vi "Tank_oneC.vi"   [LabVIEW 2012, in "Serenity_mk2.lvrbt"]
uses:
  Serenity_mk2.lvrbt
  <vilib>/NXT/Hardware/Plugins/Tetrix 180 deg Servo/Tetrix180ServoAddress.ctl
  <vilib>/NXT/Hardware/Plugins/Tetrix DC Motor/TetrixDCMotorAddress.ctl
  <vilib>/NXT/NXTIO Xnodes/NXTIONodeSubVIs/TETRIX IO Move Servos.vi
  <vilib>/FTC/FTC Calculate Drive Power - Tank.vi
  <vilib>/NXT/NXTIO Xnodes/NXTIONodeSubVIs/TETRIX IO Move DC Motors.vi
  <vilib>/NXT/NXTIO Xnodes/NXTIONodeSubVIs/TETRIX IO Check Battery.vi
  <vilib>/NXT/NXTIO Xnodes/NXTIONodeSubVIs/TETRIX IO Stop DC Motors.vi
  <vilib>/NXT/NXTIO Xnodes/AddressXNode/NXTIOAddress.xnode
  <vilib>/NXT/Subs/LVHSConnector.ctl
  <vilib>/NXT/NXTIO Xnodes/NXTIOXNode/NXTIO.xnode
  MecanumDrive/Mecanum Drive.lvrbt
  <vilib>/NXT/LegoClasses/BrickReference/BrickReference.lvclass
panel:
  # "This VI was generated based on your configuration in the Remote Control Editor. You may modify the code as needed for your robot. To test this program for an FTC match, return to the Remote Control Editor, select the \"Run Program\" tab, and choose \"Teleop\"."
types:
  T1 = typedef "Tetrix180ServoAddress.ctl" = i32
  T2 = typedef "LVHSConnector.ctl" = refnum<class "BrickReference.lvclass">
  T3 = typedef "TetrixDCMotorAddress.ctl" = i32
  T4 = cluster{"TetrixDCMotor":T3, "TetrixDCMotor 2":T3}
  T5 = typedef "FTC ControllerState.ctl" = cluster{"Left X":i8, "Left Y":i8, "Right X":i8, "Right Y":i8, "Button Encoding 9-12":u8, "Button Encoding 1-8":u8, "POV":T6}
  T6 = typedef "FTC POVState.ctl" = i8
  T7 = typedef "FTC ButtonEventType.ctl" = enum16{"Pressed", "Released"}
  T8 = cluster{"Button ID":enum16{"None", "Button 1", "Button 2", "Button 3", "Button 4", "Button 5", "Button 6", "Button 7", "Button 8", "Button 9", "Button 10", "Button 11", "Button 12", "POV Up", "POV Up Right", "POV Right", "POV Down Right", "POV Down", "POV Down Left", "POV Left", "POV Up Left"}, "Event Type":T7}[]
  T9 = typedef "FTC ButtonState.ctl" = cluster{"Button 1":bool, "Button 2":bool, "Button 3":bool, "Button 4":bool, "Button 5":bool, "Button 6":bool, "Button 7":bool, "Button 8":bool, "Button 9":bool, "Button 10":bool, "Button 11":bool, "Button 12":bool, "POV":T6}
  T10 = enum16{"None", "Button 1", "Button 2", "Button 3", "Button 4", "Button 5", "Button 6", "Button 7", "Button 8", "Button 9", "Button 10", "Button 11", "Button 12", "POV Up", "POV Up Right", "POV Right", "POV Down Right", "POV Down", "POV Down Left", "POV Left", "POV Up Left"}
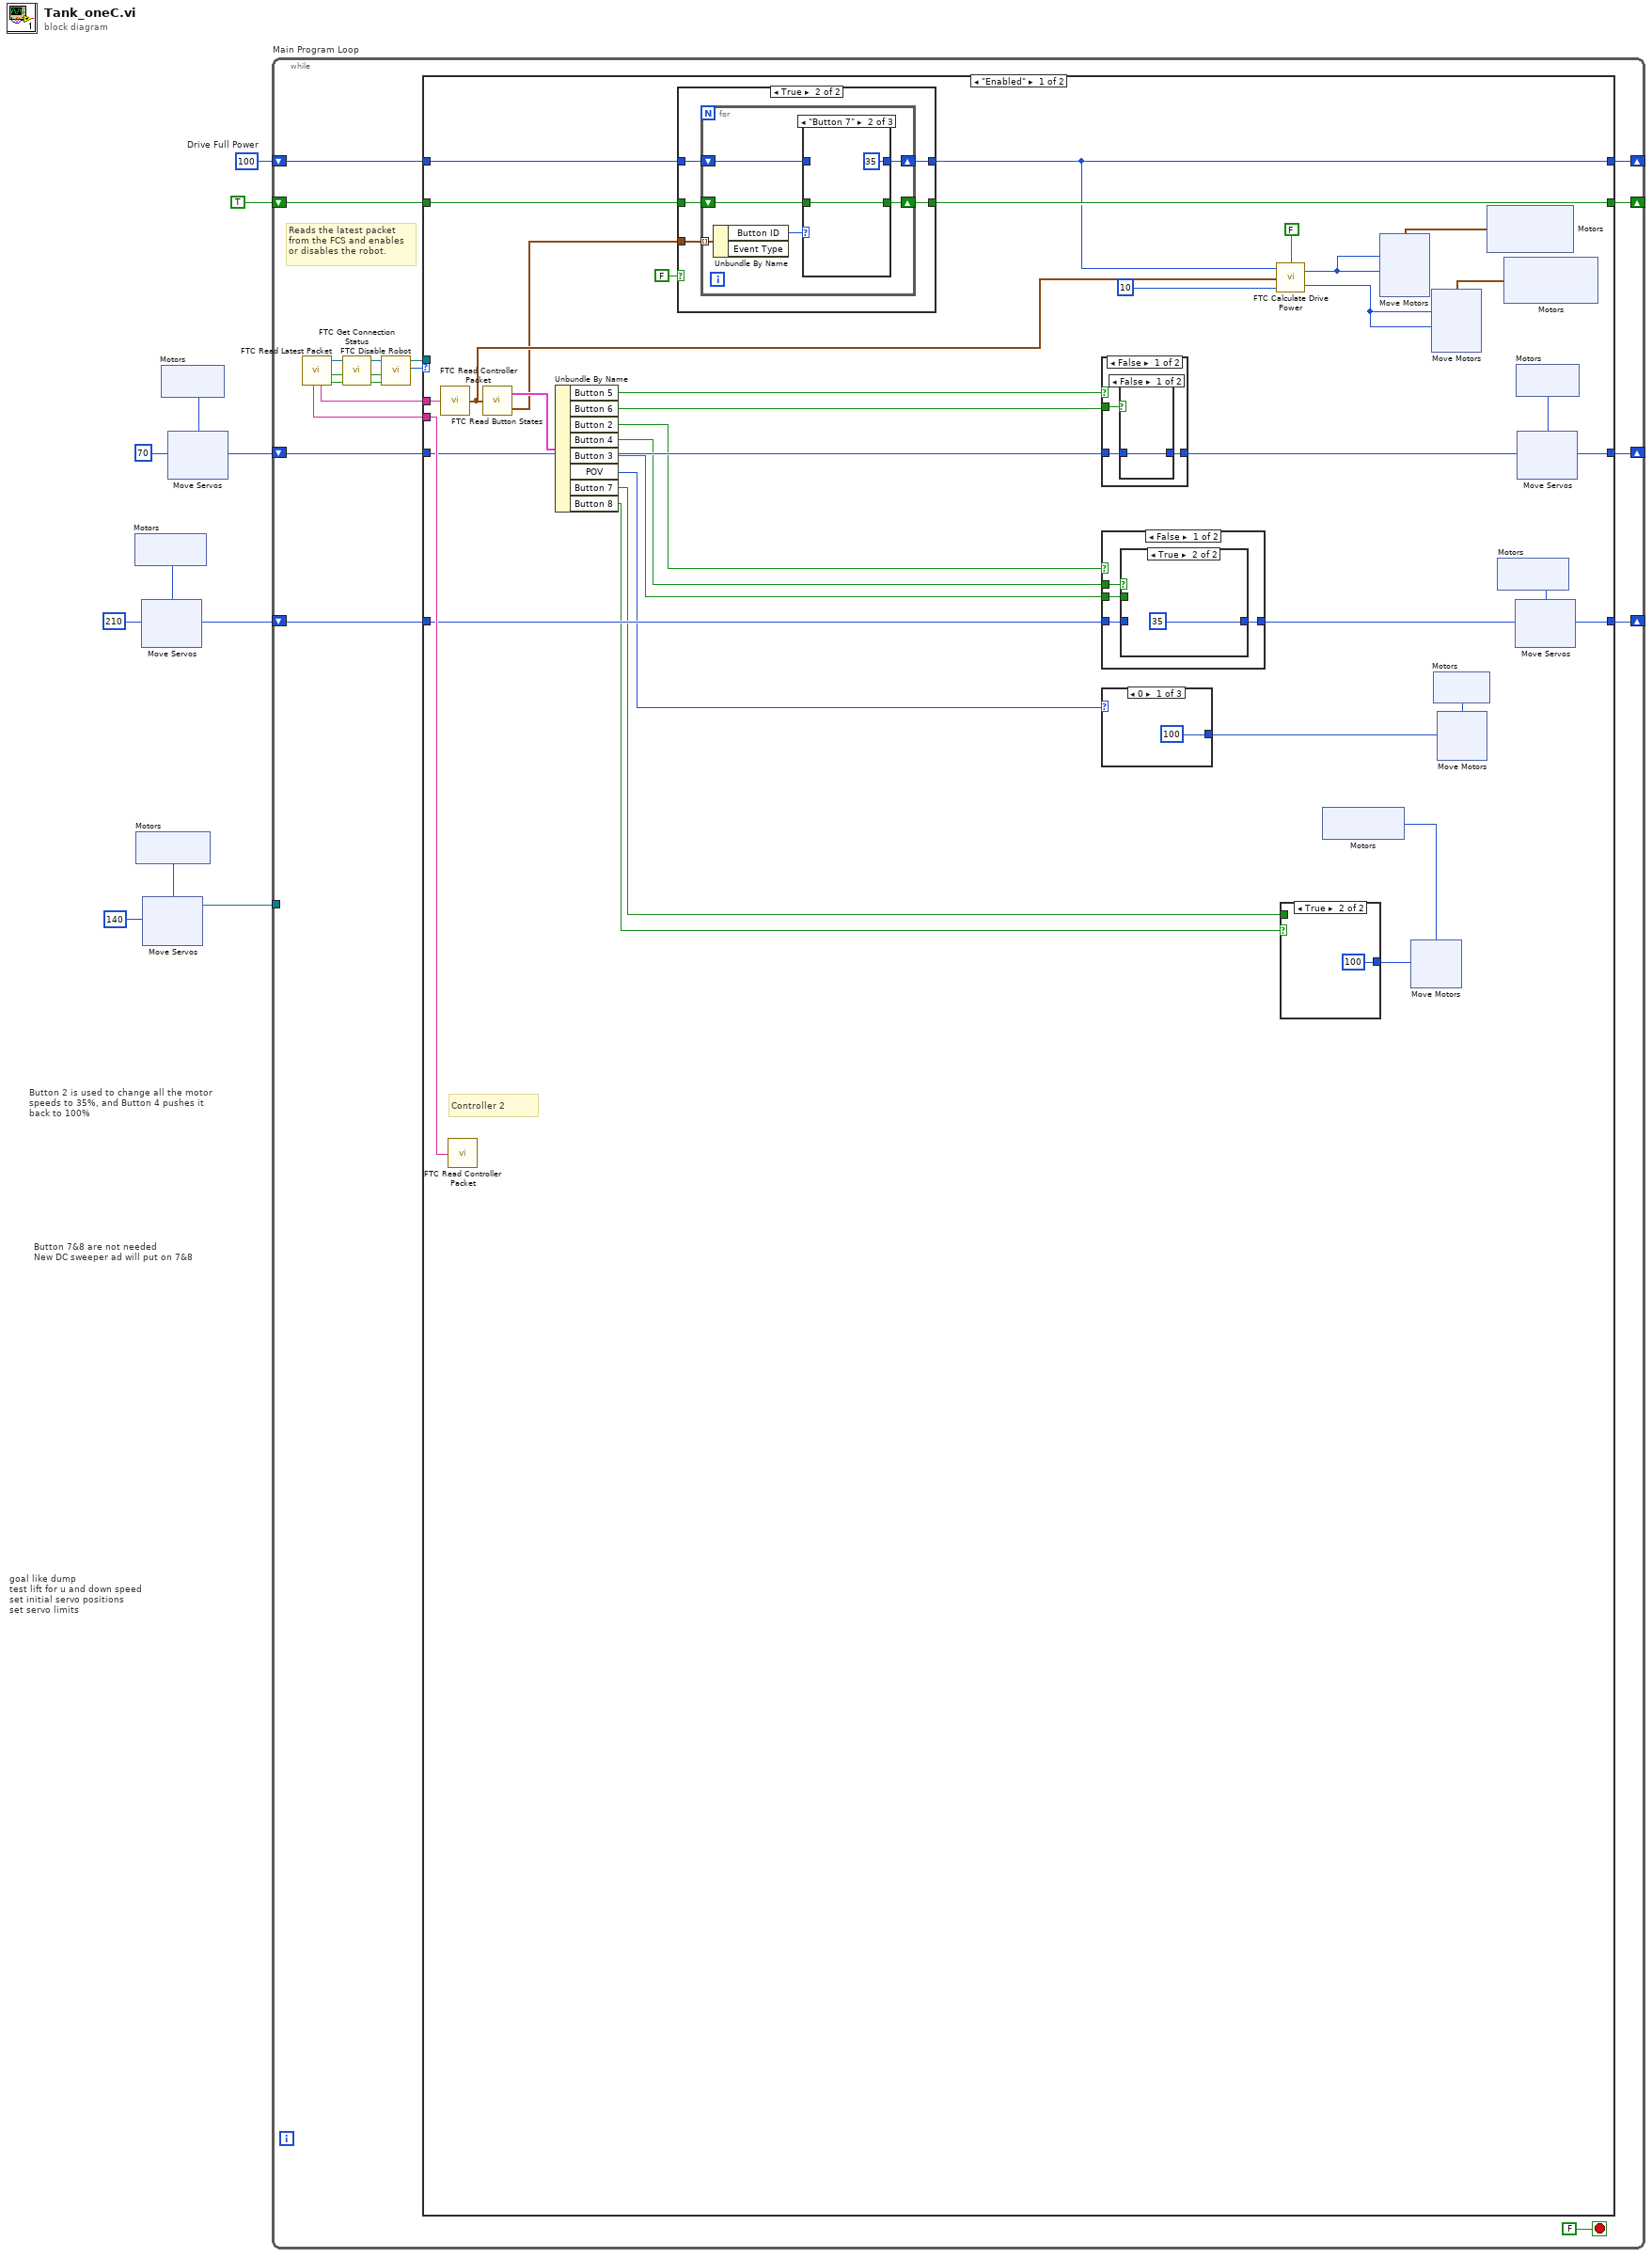
[diagram p0: block diagram]
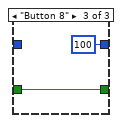
[diagram p4: hidden frame]
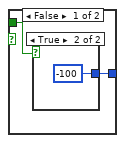
[diagram p5: hidden frame]
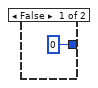
[diagram p6: hidden frame]
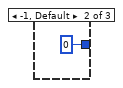
[diagram p7: hidden frame]
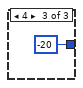
[diagram p8: hidden frame]
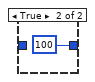
[diagram p9: hidden frame]
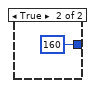
[diagram p10: hidden frame]
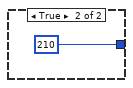
[diagram p12: hidden frame]
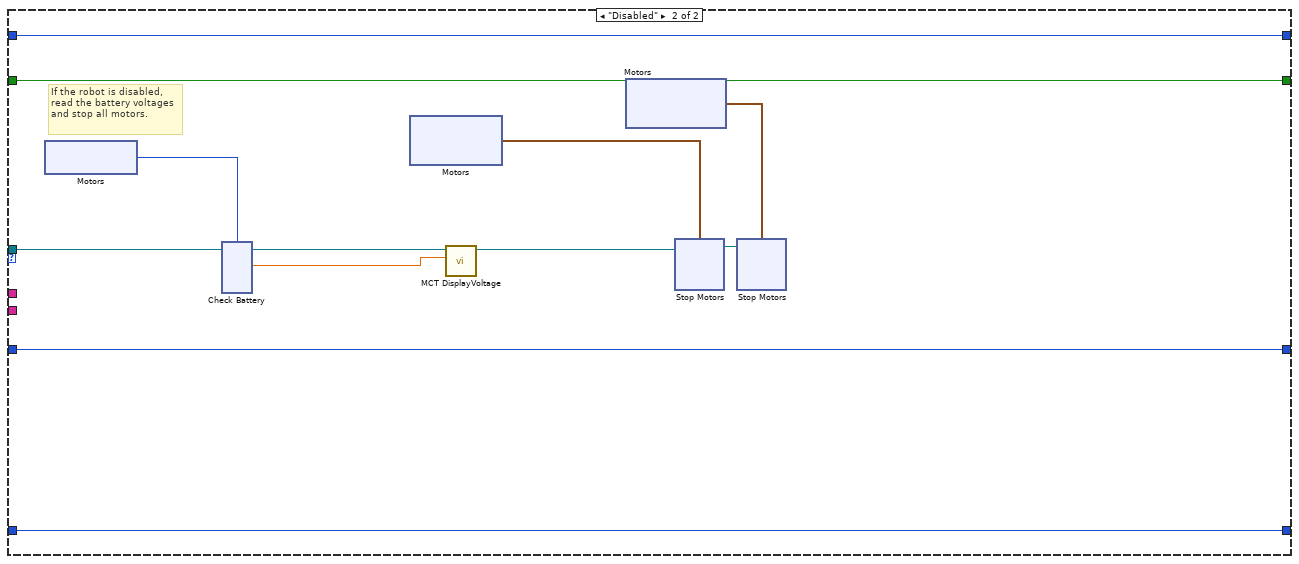
[diagram p13: hidden frame]
diagram:
  w4 = u8 210 ("Position 1")
  w6 = u8 70 ("Position 1")
  w9 = i8 100  # Drive Full Power
  # "Button 2 is used to change all the motor \nspeeds to 35%, and Button 4 pushes it \nback to 100%"
  # "goal like dump\ntest lift for u and down speed\nset initial servo positions\nset servo limits"
  # "Button 7&8 are not needed\nNew DC sweeper ad will put on 7&8"
  n1 = xnode "Motors"() -> ("Motor"=w5:T1)
  n2 = xnode "Motors"() -> ("Motor"=w3:T1)
  n3 = xnode "Move Servos"("Position 1"=w4, "Motors"=w5) -> ()  [unwired: 1 in, 1 out]
  n4 = xnode "Move Servos"("Position 1"=u8 140, "Motors"=w3) -> ("NXT/EV3"=w1:T2)  [unwired: 1 in]
  n5 = xnode "Motors"() -> ("Motor"=w7:T1)
  n6 = xnode "Move Servos"("Position 1"=w6, "Motors"=w7) -> ()  [unwired: 1 in, 1 out]
  n7 = while "Main Program Loop" {
    shift-right: [w16] -> _
    shift-left: w9 -> [w17]
    shift-right: [w14] -> _
    shift-left: TRUE -> [w15]
    shift-right: [w13] -> _
    shift-left: w6 -> [w12]
    shift-right: [w11] -> _
    shift-left: w4 -> [w10]
    tunnel: w1 -> [_]
    stop <- FALSE stop-if-true
    # "Reads the latest packet\nfrom the FCS and enables\nor disables the robot."
    n8 = call <vilib>:"FTC Read Latest Packet.vi"() -> ("Packet Received?"=w25:bool, "Stopped?"=w22:bool, "NXT"=w24:T2, "Controller 1"=w27:string, "Controller 2"=w26:string)  [unwired: 6 in, 1 out]
    n9 = call <vilib>:"FTC Get Connection Status.vi"("Packet Received?"=w25, "Stopped?"=w22, "NXT"=w24) -> ("Online?"=w19:bool, "Stopped?"=w20:bool, "NXT"=w21:T2)  [unwired: 5 in]
    n10 = call <vilib>:"FTC Disable Robot.vi"("Online?"=w19, "Stopped?"=w20, "NXT"=w21) -> ("Enabled?"=w23:enum16{"Disabled", "Enabled"}, "NXT"=w18:T2)  [unwired: 3 in]
    n11 = case "disableCase" shown="\"Enabled\"" w23 {
      tunnel: w27 -> [w62 _]
      tunnel: w26 -> [w61 _]
      tunnel: w18 -> [_ w164]
      tunnel: w17 -> [w60 w156]
      tunnel: [w50 w156] -> w16
      tunnel: w15 -> [w59 w155]
      tunnel: [w58 w155] -> w14
      tunnel: [w41 w154] -> w13
      tunnel: w12 -> [w42 w154]
      tunnel: [w46 w153] -> w11
      tunnel: w10 -> [w45 w153]
      frame "Enabled" {
        # "Controller 2"
        n12 = call <vilib>:"FTC Read Controller Packet.vi"("Packet"=w62) -> ("Controller State"=w48:T5)  [unwired: 4 in]
        n13 = call <vilib>:"FTC Read Controller Packet.vi"("Packet"=w61) -> ()  [unwired: 4 in, 1 out]
        n14 = call <vilib>:"FTC Read Button States.vi"("Controller State"=w48) -> ("Button Events"=w30:T8, "Button States"=w56:T9)  [unwired: 2 in]
        n15 = Unbundle By Name(w56) -> ("Button 5"=w44:bool, "Button 6"=w43:bool, "Button 2"=w37:bool, "Button 4"=w38:bool, "Button 3"=w39:bool, "POV"=w40:T6, "Button 7"=w32:bool, "Button 8"=w31:bool)
        n16 = case shown="True" FALSE {
          tunnel: w60 -> [w64 w69]
          tunnel: w59 -> [w63 w68]
          tunnel: [w63 w67] -> w58
          tunnel: [w64 w66] -> w50
          tunnel: w30 -> [_ w65]
          frame False {
          }
          frame True {
            n17 = for {
              tunnel: w65 -> [w75] mode=indexing
              shift-right: [w70] -> w66
              shift-left: w69 -> [w73]
              shift-right: [w71] -> w67
              shift-left: w68 -> [w72]
              n18 = Unbundle By Name(w75) -> ("Button ID"=w74:T10)  [unwired: 1 out]
              n19 = case shown="\"Button 7\"" w74 {
                tunnel: w73 -> [w76 _ _]
                tunnel: w72 -> [w77 w78 w80]
                tunnel: [w77 w78 w80] -> w71
                tunnel: [w76 i8 35 i8 100] -> w70
                frame "None", Default {
                }
                frame "Button 7" {
                }
                frame "Button 8" {
                }
              }
            }
          }
        }
        n20 = case shown="False" w44 {
          tunnel: w43 -> [w106 _]
          tunnel: w42 -> [w107 _]
          tunnel: [w108 u8 160 ("Position 1")] -> w41
          frame False {
            n21 = case shown="False" w106 {
              tunnel: [w109 u8 100 ("lower limit")] -> w108
              tunnel: w107 -> [w109 _]
              frame False {
              }
              frame True {
              }
            }
          }
          frame True {
          }
        }
        n22 = case shown="False" w37 {
          tunnel: w38 -> [w115 _]
          tunnel: [w114 u8 210] -> w46
          tunnel: w45 -> [w113 _]
          tunnel: w39 -> [w112 _]
          frame False {
            n23 = case shown="True" w115 {
              tunnel: [w116 u8 35] -> w114
              tunnel: w113 -> [w116 _]
              tunnel: w112 -> [_ _]
              frame False {
              }
              frame True {
              }
            }
          }
          frame True {
          }
        }
        n24 = case shown="0" w40 {
          tunnel: [i8 100 ("Power/Speed 1") i8 0 ("Power/Speed 1") i8 -20 ("Power/Speed 1")] -> w35
          frame 0 {
          }
          frame -1, Default {
          }
          frame 4 {
          }
        }
        n25 = call-poly <vilib>:"FTC Calculate Drive Power.vi"("Reverse"=FALSE, "Deadband (10)"=i8 10, "Controller State"=w48, "Power Level (50)"=w50) -> ("Right Motor Power"=w49:i8, "Left Motor Power"=w51:i8)
        n26 = case shown="True" w31 {
          tunnel: w32 -> [w91 _]
          tunnel: [w90 i8 100] -> w34
          frame False {
            n27 = case shown="True" w91 {
              tunnel: [i8 0 i8 -100] -> w90
              frame False {
              }
              frame True {
              }
            }
          }
          frame True {
          }
        }
        n28 = xnode "Motors"() -> ("Motor"=w33:T3)
        n29 = xnode "Move Motors"("Power/Speed 1"=w34, "Motors"=w33) -> ()  [unwired: 1 in, 1 out]
        n30 = xnode "Motors"() -> ("Motor"=w36:T3)
        n31 = xnode "Move Motors"("Power/Speed 1"=w35, "Motors"=w36) -> ()  [unwired: 1 in, 1 out]
        n32 = xnode ("Motors")() -> ("Motor"=w52:cluster{"TetrixDCMotor":T3, "TetrixDCMotor":T3})
        n33 = xnode ("Move Motors")("Power/Speed 2"=w51, "Power/Speed 1"=w51, "Motors"=w52) -> ()  [unwired: 1 in, 1 out]
        n34 = xnode "Motors"() -> ("Motor"=w47:T1)
        n35 = xnode ("Motors")() -> ("Motor"=w53:cluster{"TetrixDCMotor":T3, "TetrixDCMotor":T3})
        n36 = xnode ("Move Motors")("Power/Speed 2"=w49, "Power/Speed 1"=w49, "Motors"=w53) -> ()  [unwired: 1 in, 1 out]
        n37 = xnode "Move Servos"("Position 1"=w46, "Motors"=w47) -> ()  [unwired: 1 in, 1 out]
        n38 = xnode "Motors"() -> ("Motor"=w57:T1)
        n39 = xnode "Move Servos"("Position 1"=w41, "Motors"=w57) -> ()  [unwired: 1 in, 1 out]
      }
      frame "Disabled" {
        # "If the robot is disabled, read the battery voltages and stop all motors."
        n40 = xnode ("Motors")() -> ("Motor"=w163:T3)
        n41 = xnode ("Check Battery")("Motors"=w163, "NXT/EV3"=w164) -> ("Voltage 1"=w162:sgl, "NXT/EV3"=w161:T2)
        n42 = xnode "Motors"() -> ("Motor"=w160:cluster{"TetrixDCMotor":T3, "TetrixDCMotor":T3})
        n43 = call <vilib>:"MCT DisplayVoltage.vi"("Motor Voltage"=w162, "NXT"=w161) -> ("NXT"=w159:T2)  [unwired: 9 in]
        n44 = xnode "Motors"() -> ("Motor"=w158:cluster{"TetrixDCMotor":T3, "TetrixDCMotor":T3})
        n45 = xnode "Stop Motors"("Motors"=w160, "NXT/EV3"=w159) -> ("NXT/EV3"=w157:T2)
        n46 = xnode "Stop Motors"("Motors"=w158, "NXT/EV3"=w157) -> ()  [unwired: 1 out]
      }
    }
  }
